vi "Task1AA Not SubVI.vi"() -> ()   [LabVIEW 2016]
panel:
  out "g, acceleration due to gravity":dbl
  in  "r, radius (m)":dbl
  in  "m, mass (kg)":dbl
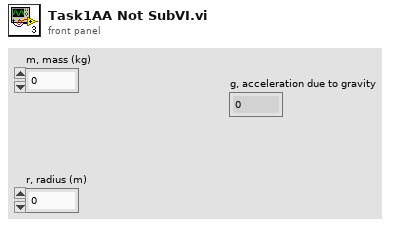
[diagram p1: front panel]
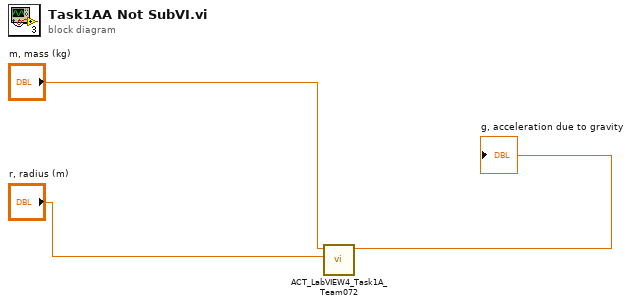
[diagram p0: block diagram]
diagram:
  n1 = call "ACT_LabVIEW4_Task1A_Team072.vi"("r, radius (m)"="r, radius (m)", "m, mass (kg)"="m, mass (kg)") -> ("g, acceleration due to gravity"=→"g, acceleration due to gravity":dbl)  [unwired: 9 in]
